vi "Pre Launch Init.vi"(11 "RDS Test Child in":refnum<class "RDS Test Child.lvclass">) -> (0 "error out":errorcluster, 3 "RDS Test Child out":refnum<class "RDS Test Child.lvclass">)   [LabVIEW 2015, in "RDS Test Child.lvlib" / "RDS Test Child.lvclass"]
doc: "(<B>Filename</B>: Actor Framework.lvlib:Actor.lvclass:Pre Launch Init.vi)\n\nDefines behavior that occurs after the Launch Nested Actor method is invoked but before the actor's Actor Core method begins running.\n\nBy default, this method does nothing. A descendant class may override it to define behavior."
uses:
  RDS Test Child.lvclass
  RDS Parent Actor/RDS Parent Actor/RDS Parent Actor.lvclass/RDS Parent Actor.ctl
  RDS Parent Actor/RDS Parent Actor/RDS Parent Actor.lvclass
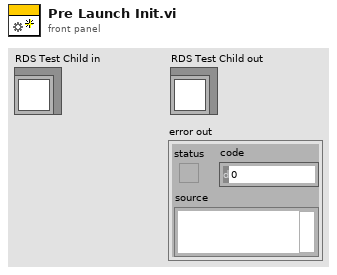
[diagram p1: front panel]
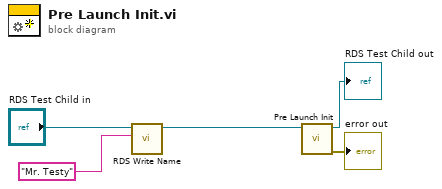
[diagram p0: block diagram]
diagram:
  n1 = call "RDS Write Name.vi"("Name"="Mr. Testy", "RDS Parent Actor in"="RDS Test Child in") -> ("RDS Parent Actor out"=w2:refnum<class "RDS Test Child.lvclass">)  [unwired: 8 in, 1 out]
  n2 = call-parent "Pre Launch Init.vi"("Actor in"=w2) -> ("error out"=→"error out":errorcluster, "Actor out"=→"RDS Test Child out":refnum<class "RDS Test Child.lvclass">)  [unwired: 9 in]
